vi "M937X Initialize and Config.vi"(8 "error in (no error)":errorcluster {"code" format="%.0x"}, 11 "NETAN":refnum<k15> caption="resource string") -> (0 "error out":errorcluster {"code" format="%.0x"}, 3 "instrument handle out":refnum<k15>)   [LabVIEW 2015]
uses:
  <instrlib>/Agilent NA/Agilent NA.lvlib
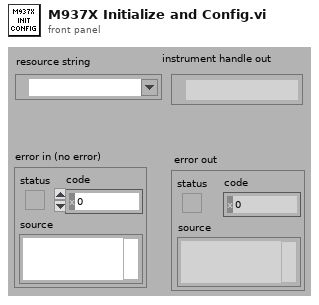
[diagram p1: front panel]
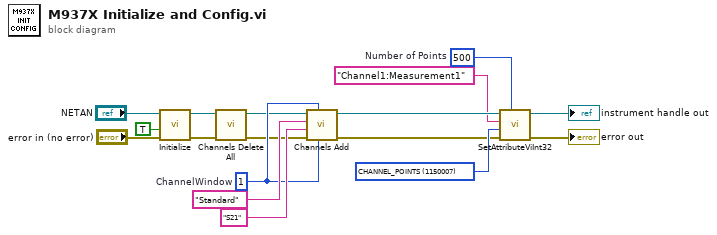
[diagram p0: block diagram]
diagram:
  w4 = 500  # Number of Points
  w12 = 1  # ChannelWindow
  w13 = u32 1150007 items=["CHANNEL_AVERAGING_FACTOR"=1150002, "CHANNEL_MEASUREMENT_ELECTRICAL_DELAY_MEDIUM"=1150178, "CHANNEL_MEASUREMENT_ELECTRICAL_DELAY_UNITS"=1150175, "CHANNEL_MEASUREMENT_FORMAT"=1150014, "CHANNEL_MEASUREMENT_LIMIT_NUMBER"=1150020, "CHANNEL_MEASUREMENT_TIME_DOMAIN_GATING_SHAPE"=1150140, "CHANNEL_MEASUREMENT_TIME_DOMAIN_GATING_TYPE"=1150144, "CHANNEL_MEASUREMENT_TIME_DOMAIN_PARAMETERS"=1150137, "CHANNEL_MEASUREMENT_TIME_DOMAIN_TRANSFORM_MODE"=1150147, "CHANNEL_MEASUREMENT_TRACE_MATH"=1150017, "CHANNEL_POINTS"=1150007, "CHANNEL_SWEEP_MODE"=1150009, "CHANNEL_SWEEP_TYPE"=1150012, "CHANNEL_TRIGGER_MODE"=1150013, "DISPLAY_ARRANGE_WINDOWS"=1150181, "SYSTEM_TIME_OUT_MILLISECONDS"=1150040, "TRIGGER_SOURCE"=1150042, "WINDOW_SIZE"=1150133, "WINDOW_TABLE"=1150134] ("AttributeID")
  n1 = call <instrlib>:"Initialize.vi"("error in (no error)"="error in (no error)", "reset device (Off)"=TRUE, "resource name"="NETAN") -> ("error out"=w7:errorcluster, "instrument handle out"=w8:refnum<k15>)  [unwired: 7 in]
  n2 = call <instrlib>:"Channels Delete All.vi"("error in (no error)"=w7, "instrument handle"=w8) -> ("error out"=w6:errorcluster, "instrument handle out"=w5:refnum<k15>)  [unwired: 8 in]
  n3 = call <instrlib>:"Channels Add.vi"("WindowNumber"=w12, "ChannelNumber"=w12, "error in (no error)"=w6, "ChannelParameter"="S21", "ChannelType"="Standard", "instrument handle"=w5) -> ("error out"=w10:errorcluster, "instrument handle out"=w11:refnum<k15>)  [unwired: 3 in, 1 out]
  n4 = call <instrlib>:"SetAttributeViInt32.vi"("AttributeValue"=w4, "error in (no error)"=w10, "AttributeID"=w13, "RepCapIdentifier"="Channel1:Measurement1", "instrument handle"=w11) -> ("error out"=→"error out":errorcluster, "instrument handle out"=→"instrument handle out":refnum<k15>)  [unwired: 5 in]
